vi "OpenTDMS.vi"(10 "Name in":string, 11 "FilesPath":path) -> (2 "Name out":string, 3 "Path":path)   [LabVIEW 2019]
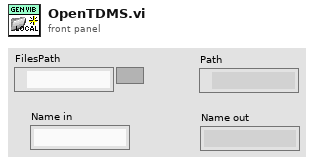
[diagram p1: front panel]
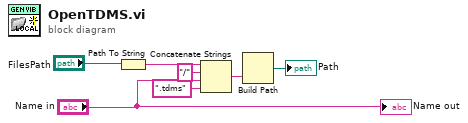
[diagram p0: block diagram]
diagram:
  n1 = Path To String(path="FilesPath") -> (string=w3:string)
  n2 = Concatenate Strings(w3, "/" ("string"), "Name in", ".tdms" ("string")) -> (w6:string)
  n3 = Build Path(name or relative path=w6) -> (appended path=→"Path":path)  [unwired: 1 in]
  "Name out" <- "Name in"
